vi "Exercise9.3-FM_USRP_TX.vi"() -> ()   [LabVIEW 2013]
uses:
  <vilib>/sound2/lvsound2.llb/Sound File Info (path).vi
  <vilib>/sound2/lvsound2.llb/Sound File Read Open.vi
  <vilib>/Analysis/2dsp.llb/Rational Resample (single channel, DBL).vi
  <vilib>/sound2/lvsound2.llb/Sound File Read (DBL).vi
  <instrlib>/niUSRP/niUSRP Write Tx Data (CDB).vi
  <vilib>/Analysis/NI_AALPro.lvlib
panel:
  out "Constellation":cluster{dbl[], dbl[]}(graph)
  out "Output waveform":waveform(dbl)(graph)
  out "coerced gain":dbl format="%#_6f"
  out "coerced IQ rate":dbl=100000.0 format="%#_6p"
  out "coerced carrier frequency":dbl=100000.0 format="%#_6p"
  in  "number of samples":i32=10000
  in  "IQ rate":dbl=200000.0 format="%#_6p"
  in  "carrier frequency":dbl=2400000000.0 format="%#_6p"
  in  "Gain":dbl
  in  "FM deviation (Hz)":dbl(slide)=75000.0 scale=0.0..100000.0
  in  "active antenna":string="TX1"
  in  "stop":bool
  in  "path":path=path "D:/File/let it go.wav"
  in  "IP":refnum<k15>="192.168.10.2"
  out "error out":errorcluster
  # "FM Transmitter"
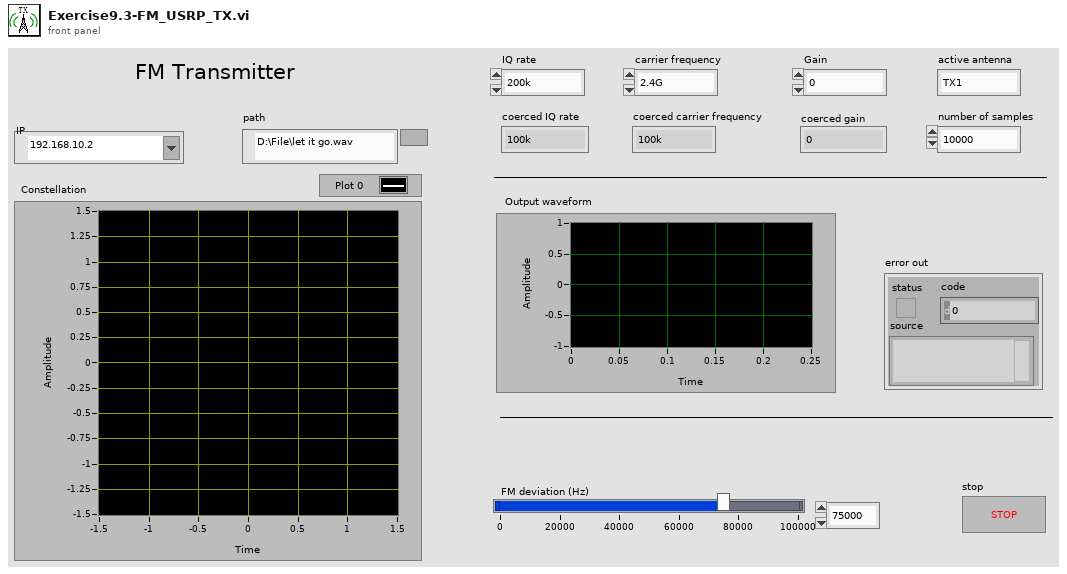
[diagram p1: front panel]
types:
  T1 = typedef "Sound Data Format.ctl" = cluster{"sample rate (S/s)":dbl, "number of channels":i32, "bits per sample":i32}
  T2 = typedef "Sound File Refnum.ctl" = refnum<file>
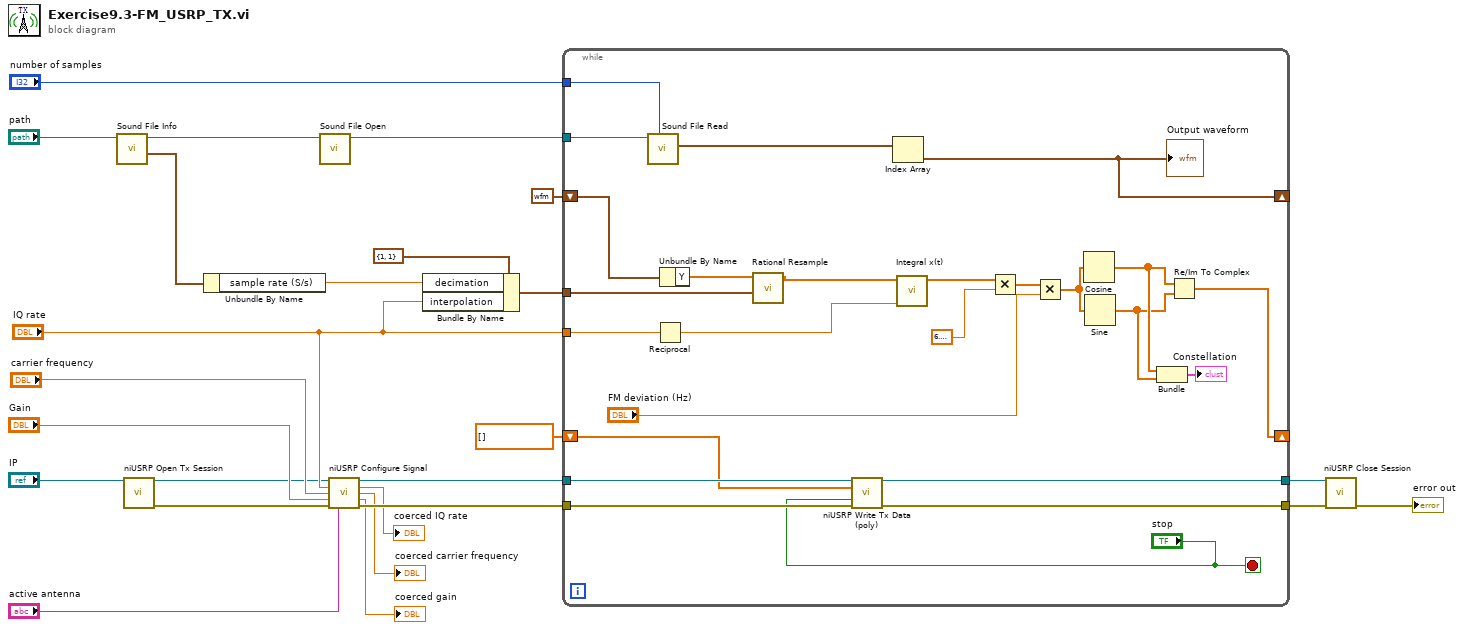
[diagram p0: block diagram]
diagram:
  n1 = call-poly <vilib>:"Sound File Info.vi"("path"="path") -> ("sound format"=w9:T1, "path out"=w20:path)  [unwired: 7 in, 2 out]
  n2 = call <instrlib>:"niUSRP Open Tx Session.vi"("device names"="IP") -> ("session handle out"=w3:refnum<k15>, "error out"=w1:errorcluster)  [unwired: 13 in]
  n3 = Unbundle By Name(w9) -> ("sample rate (S/s)"=w7:dbl)
  n4 = call-poly <vilib>:"Sound File Open.vi"("path"=w20) -> ("sound file refnum"=w13:T2)  [unwired: 9 in, 1 out]
  n5 = call <instrlib>:"niUSRP Configure Signal.vi"("session handle"=w3, "IQ rate"="IQ rate", "carrier frequency"="carrier frequency", "gain"="Gain", "error in (no error)"=w1, "active antenna"="active antenna") -> ("session handle out"=w21:refnum<k15>, "coerced IQ rate"=→"coerced IQ rate":dbl, "coerced carrier frequency"=→"coerced carrier frequency":dbl, "coerced gain"=→"coerced gain":dbl, "error out"=w23:errorcluster)  [unwired: 5 in]
  n6 = Bundle By Name(cluster=cluster{"interpolation":i32, "decimation":i32} {"interpolation"=1, "decimation"=1} ("resample factor"), "decimation"=w7, "interpolation"="IQ rate") -> (w10:cluster{"interpolation":i32, "decimation":i32})
  n7 = while {
    tunnel: w21 -> [w50]
    tunnel: [w49] -> w25
    tunnel: [w48] -> w24
    tunnel: w23 -> [w47]
    tunnel: "IQ rate" -> [w34]
    tunnel: w13 -> [w42]
    tunnel: "number of samples" -> [w41]
    tunnel: w10 -> [w33]
    shift-right: [w29] -> _
    shift-left: waveform(dbl) {"t0"=timestamp(0 s since 1904-01-01), "dt"=1.0, "Y"=[]} ("data") -> [w32]
    shift-right: [w31] -> _
    shift-left: cdb[] [] -> [w30]
    stop <- "stop" stop-if-true
    n8 = call-poly <vilib>:"Sound File Read.vi"("number of samples/ch (-1: all)"=w41, "sound file refnum"=w42) -> ("data"=w40:waveform(dbl)[])  [unwired: 5 in, 4 out]
    n9 = Reciprocal(x=w34) -> (1/x=w38:dbl)
    n10 = Unbundle By Name(w32) -> ("Y"=w37:dbl[])
    n11 = call-poly <vilib>:"Rational Resample.vi"("resample factor"=w33, "X"=w37) -> ("Y"=w36:dbl[])  [unwired: 7 in, 2 out]
    n12 = call-poly <instrlib>:"niUSRP Write Tx Data (poly).vi"("session handle"=w50, "data"=w30, "end of data?"="stop", "error in (no error)"=w47) -> ("session handle out"=w49:refnum<k15>, "error out"=w48:errorcluster)  [unwired: 10 in]
    n13 = Index Array(array=w40) -> (element=w29:waveform(dbl))  [unwired: 1 in]
    "Output waveform" <- w29
    n14 = call <vilib>:"Integral x(t).vi"("dt"=w38, "X"=w36) -> ("Integral X"=w39:dbl[])  [unwired: 8 in, 1 out]
    n15 = Multiply(x=w39, y=6.283185307179586) -> (x*y=w45:dbl[])
    n16 = Multiply(x=w45, y="FM deviation (Hz)") -> (x*y=w46:dbl[])
    n17 = Cosine(x=w46) -> (cos(x)=w28:dbl[])
    n18 = Sine(x=w46) -> (sin(x)=w27:dbl[])
    n19 = Bundle(w28, w27) -> (→"Constellation":cluster{dbl[], dbl[]})  [unwired: 1 in]
    n20 = Re/Im To Complex(1:w27, 2:w28) -> (0:w31:cdb[])
  }
  n21 = call <instrlib>:"niUSRP Close Session.vi"("session handle"=w25, "error in (no error)"=w24) -> ("error out"=→"error out":errorcluster)  [unwired: 13 in]
